vi "Stop Temperature.vi"(0 "reference in":refnum<class "Temp.lvclass">, 5 "error in (no error)":errorcluster) -> (14 "reference out":refnum<class "Temp.lvclass">, 19 "error out":errorcluster)   [LabVIEW 2017, in "Temp.lvclass"]
uses:
  Temp.lvclass
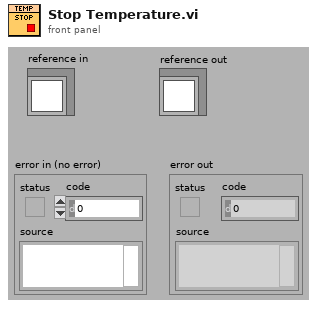
[diagram p1: front panel]
types:
  T1 = typedef "Temp.lvclass/ObjectAttributes.ctl" = cluster{"Temperature Task":refnum<k21>, "Temperature Readings":dbl[], "Thermocouple Type":i32, "Temperature Units":i32, "Average Temperature":dbl, "Number of Temperature Modules":i32, "Number of Total Temperature Channels":i32, "Temperature On/Off Status":bool, "Temperature Module Names (NI-Max Name)":string[], "Number of Channels Per Temperature  Module":i32[], "Temperature VI Reference":refnum<vi>}
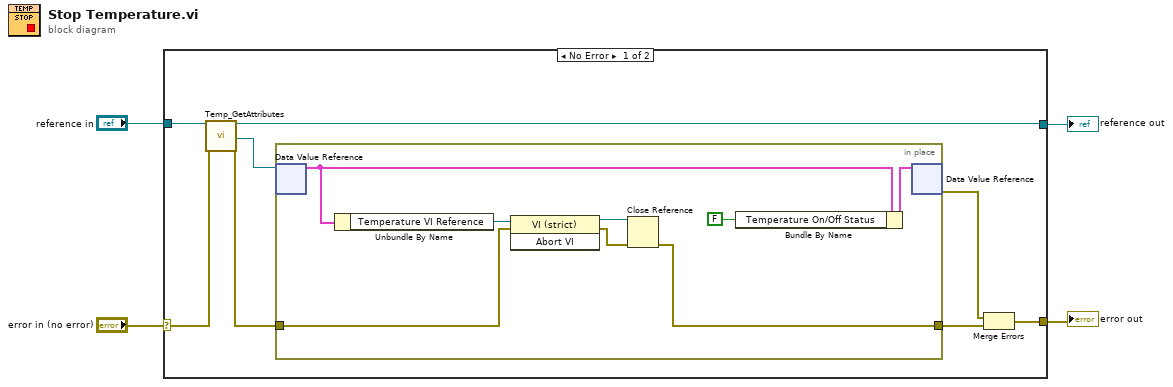
[diagram p0: block diagram]
diagram:
  n1 = case shown="No Error" "error in (no error)" {
    selector: "error in (no error)" -> [w11 w22]
    tunnel: [w8 w22] -> w3
    tunnel: [w9 w21] -> w1
    tunnel: "reference in" -> [w12 w21]
    frame No Error {
      n2 = call "Temp_GetAttributes.vi"("reference in"=w12, "error in (no error)"=w11) -> ("reference out"=w9:refnum<class "Temp.lvclass">, "DataRef"=w7:refnum<data-value>, "error out"=w6:errorcluster)  [unwired: 14 in, 1 out]
      n3 = in-place {
        in-place-border: w6 -> [w14]
        in-place-border: [w13] -> w5
        n4 = in-place-dvr #1(w7) -> (w19:T1)  [unwired: 1 out]
        n5 = Unbundle By Name(w19) -> ("Temperature VI Reference"=w17:refnum<vi>)
        n6 = invoke class="VI (strict)" method="Abort VI"(reference=w17, error in=w14) -> (reference out=w16:refnum<vi>, error out=w15:errorcluster)  [unwired: 1 in, 1 out]
        n7 = Close Reference(reference=w16, error in (no error)=w15) -> (error out=w13:errorcluster)
        n8 = Bundle By Name(cluster=w19, "Temperature On/Off Status"=FALSE) -> (w20:T1)
        n9 = in-place-dvr #1(w20) -> (w10:errorcluster)  [unwired: 1 out]
      }
      n10 = Merge Errors(w10, w5) -> (w8:errorcluster)
    }
    frame Error {
    }
  }
  "error out" <- w3
  "reference out" <- w1
